vi "~ simulation prototype.vi"() -> ()   [LabVIEW 2017]
panel:
  in  "stop":bool
  out "Boolean":bool
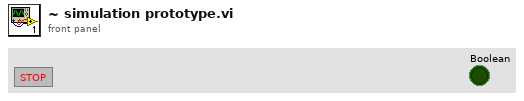
[diagram p1: front panel]
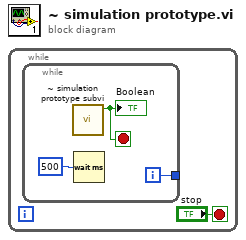
[diagram p0: block diagram]
diagram:
  n1 = while {
    stop <- "stop" stop-if-true
    n2 = while {
      tunnel: [w2] -> _
      i -> [w2]
      stop <- w4 stop-if-true
      n3 = call "~ simulation prototype subvi.vi"() -> ("Motion Stopped = T"=w4:bool)  [unwired: 11 in]
      "Boolean" <- w4
      n4 = Wait (ms)(milliseconds to wait=u32 500) -> ()  [unwired: 1 out]
    }
  }
